vi "Solution part 2.vi"() -> ()   [LabVIEW 2020]
panel:
  out "result":u64
  in  "data?":bool
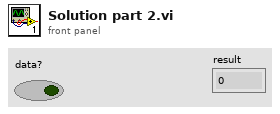
[diagram p1: front panel]
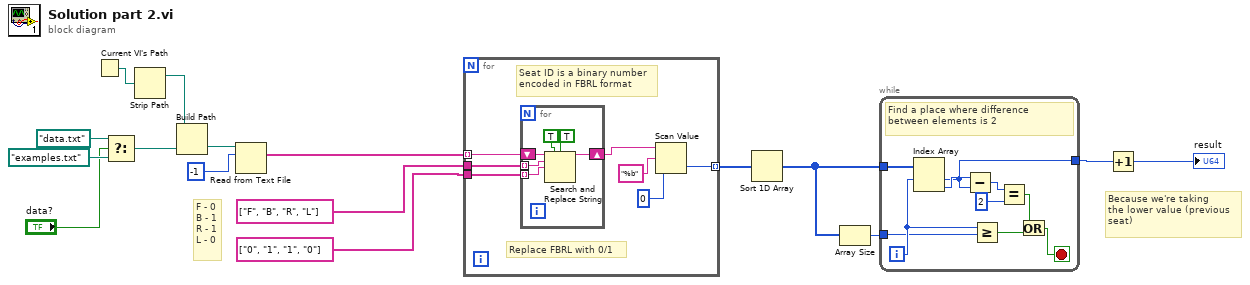
[diagram p0: block diagram]
diagram:
  # "Because we're taking\nthe lower value (previous\nseat)"
  # "F - 0\nB - 1\nR - 1\nL - 0"
  n1 = Current VI's Path() -> (path=w12:path)
  n2 = Select(t=path "data.txt", s="data?", f=path "examples.txt") -> (s? t:f=w13:path)
  n3 = Strip Path(path=w12) -> (stripped path=w11:path)  [unwired: 1 out]
  n4 = Build Path(base path=w11, name or relative path=w13) -> (appended path=w10:path)
  n5 = Read from Text File(file (use dialog)=w10, count=-1) -> (text=w8:string[])  [unwired: 2 in, 3 out]
  n6 = for {
    tunnel: w8 -> [w23] mode=indexing
    tunnel: [w18] -> w5 mode=indexing
    tunnel: string[] ["F", "B", "R", "L"] -> [w22]
    tunnel: string[] ["0", "1", "1", "0"] -> [w21]
    # "Seat ID is a binary number\nencoded in FBRL format"
    # "Replace FBRL with 0/1"
    n7 = for {
      shift-right: [w28] -> w19
      shift-left: w23 -> [w29]
      tunnel: w22 -> [w27] mode=indexing
      tunnel: w21 -> [w26] mode=indexing
      n8 = Search and Replace String(replace all?=TRUE ("replace all? (F)"), case sensitive?=TRUE ("ignore case? (F)"), input string=w29, search string=w27, replace string=w26) -> (result string=w28:string)  [unwired: 3 in, 3 out]
    }
    n9 = Scan Value(string=w19, format string="%b", default (0 dbl)=u64 0) -> (value=w18:u64)  [unwired: 1 out]
  }
  n10 = Sort 1D Array(array=w5) -> (sorted array=w2:u64[])
  n11 = Array Size(array=w2) -> (size(s)=w1:i32)
  n12 = while {
    tunnel: w2 -> [w39]
    tunnel: [w34] -> w4
    tunnel: w1 -> [w32]
    i -> [w33]
    stop <- w31 stop-if-true
    # "Find a place where difference between elements is 2"
    n13 = Index Array(array=w39, index #1=w33) -> (element #1=w34:u64, element #2=w37:u64)  [unwired: 1 in]
    n14 = Subtract(x=w37, y=w34) -> (x-y=w38:u64)
    n15 = Greater Or Equal?(x=w33, y=w32) -> (x >= y?=w30:bool)
    n16 = Equal?(x=w38, y=u64 2) -> (x = y?=w35:bool)
    n17 = Or(x=w35, y=w30) -> (x .or. y?=w31:bool)
  }
  n18 = Increment(x=w4) -> (x+1=→"result":u64)
